vi "detach_observer.vi"(8 "error in (no error)":errorcluster, 10 "top-level component type":T1, 11 "GenericToplevelComponent in":refnum<class "GenericToplevelComponent.lvclass">) -> (0 "error out":errorcluster, 3 "GenericToplevelComponent out":refnum<class "GenericToplevelComponent.lvclass">)   [LabVIEW 2010, in "GenericToplevelComponent.lvclass"]
uses:
  GenericToplevelComponent.lvclass
  enumerations/top-level_component_type_enum.ctl
  GenericToplevelComponent.lvclass/GenericToplevelComponent.ctl
  GenericComponent/GenericComponent/GenericComponent.lvclass
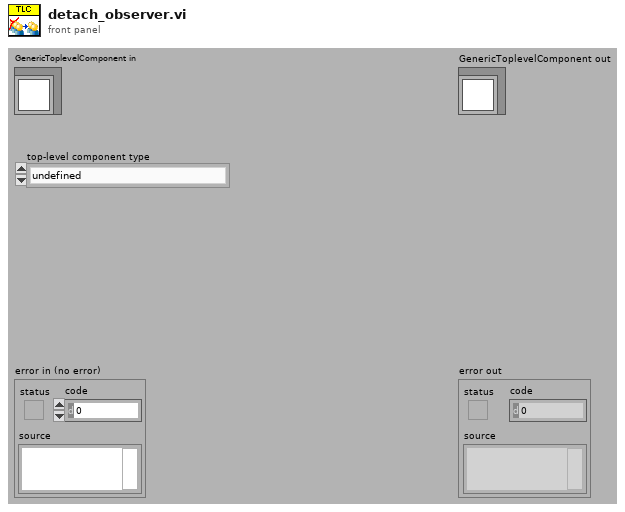
[diagram p1: front panel]
types:
  T1 = typedef "top-level_component_type_enum.ctl" = enum16{"undefined", "ImagingMode", "ScanHead", "DAQ", "ImageAssembler", "Display", "DataCollection", "Analyser", "Stimulator", "ExperimentController", "Instrument", "Stage"}
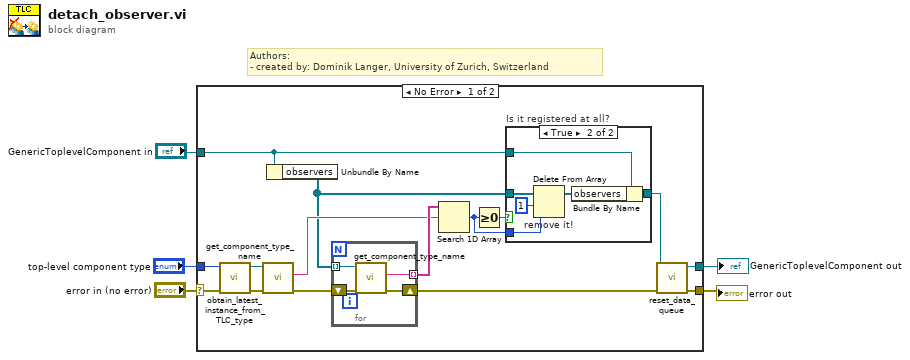
[diagram p0: block diagram]
diagram:
  # "Authors: \n- created by: Dominik Langer, University of Zurich, Switzerland"
  n1 = case shown="No Error" "error in (no error)" {
    selector: "error in (no error)" -> [w9 w33]
    tunnel: [w12 w33] -> w3
    tunnel: [w10 w32] -> w2
    tunnel: "GenericToplevelComponent in" -> [w16 w32]
    tunnel: "top-level component type" -> [w6 _]
    frame No Error {
      n2 = call "obtain_latest_instance_from_TLC_type.vi"("error in (no error)"=w9, "top-level component type"=w6) -> ("error out"=w8:errorcluster, "GenericToplevelComponent.lvclass"=w7:refnum<class "GenericToplevelComponent.lvclass">)  [unwired: 8 in]
      n3 = call-dynamic "get_component_type_name.vi"("error in (no error)"=w8, "GenericPlugin in"=w7) -> ("error out"=w19:errorcluster, "component type"=w18:string)  [unwired: 7 in, 1 out]
      n4 = Unbundle By Name(w16) -> ("observers"=w17:refnum<class "GenericComponent.lvclass">[])
      n5 = for {
        shift-right: [w30] -> w13
        shift-left: w19 -> [w31]
        tunnel: w17 -> [w29] mode=indexing
        tunnel: [w28] -> w20 mode=indexing
        n6 = call-dynamic "get_component_type_name.vi"("error in (no error)"=w31, "GenericPlugin in"=w29) -> ("error out"=w30:errorcluster, "component type"=w28:string)  [unwired: 7 in, 1 out]
      }
      n7 = Search 1D Array(1D array=w20, element=w18) -> (index of element=w14:i32)  [unwired: 1 in]
      n8 = Greater Or Equal To 0?(x=w14) -> (x >= 0?=w15:bool)
      n9 = case "Is it registered at all?" shown="True" w15 {
        tunnel: w17 -> [_ w27]
        tunnel: w16 -> [w21 w25]
        tunnel: [w21 w24] -> w11
        tunnel: w14 -> [_ w23]
        frame False {
          # "No action required..."
        }
        frame True {
          n10 = Delete From Array "remove it!"(array=w27, length=1, index=w23) -> (array with subset deleted=w26:refnum<class "GenericComponent.lvclass">[])  [unwired: 1 out]
          n11 = Bundle By Name(cluster=w25, "observers"=w26) -> (w24:refnum<class "GenericToplevelComponent.lvclass">)
        }
      }
      n12 = call-dynamic "reset_data_queue.vi"("error in (no error)"=w13, "GenericToplevelComponent in"=w11) -> ("error out"=w12:errorcluster, "GenericToplevelComponent out"=w10:refnum<class "GenericToplevelComponent.lvclass">)  [unwired: 8 in]
    }
    frame Error {
    }
  }
  "error out" <- w3
  "GenericToplevelComponent out" <- w2
